vi "Close.vi"(8 "error in":errorcluster, 11 "NI 9862 in":refnum<class "NI 9862.lvclass">) -> (0 "error out":errorcluster, 3 "NI 9862 out":refnum<class "NI 9862.lvclass">)   [LabVIEW 2024, in "NI 9862.lvclass"]
uses:
  NI 9862.lvclass
  NI 9862.lvclass/NI 9862.ctl
  Source/Interfaces/IConfigure/IStoreConfiguration.lvclass
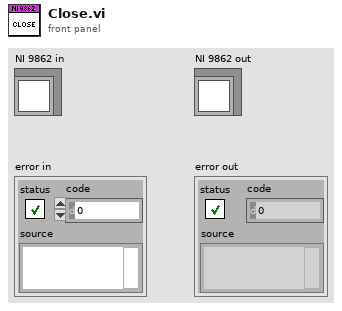
[diagram p1: front panel]
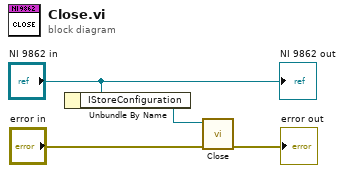
[diagram p0: block diagram]
diagram:
  n1 = Unbundle By Name("NI 9862 in") -> ("IStoreConfiguration"=w1:refnum<class "IStoreConfiguration.lvclass">)
  n2 = call-dynamic "Close.vi"("error in"="error in", "IStoreConfiguration in"=w1) -> ("error out"=→"error out":errorcluster)  [unwired: 8 in, 1 out]
  "NI 9862 out" <- "NI 9862 in"
